vi "Day07-03_디지털 신호 제어.vi"() -> ()   [LabVIEW 2021]
uses:
  <vilib>/DAQmx/create/channels.llb/DAQmx Create Channel (DI-Digital Input).vi
  <vilib>/DAQmx/create/channels.llb/DAQmx Create Channel (DO-Digital Output).vi
  <vilib>/DAQmx/write.llb/DAQmx Write (Digital U8 1Chan 1Samp).vi
  <vilib>/DAQmx/read.llb/DAQmx Read (Digital 1D Bool 1Chan 1Samp).vi
  <vilib>/DAQmx/read.llb/DAQmx Read (Digital U8 1Chan 1Samp).vi
  <vilib>/DAQmx/read.llb/DAQmx Read (Analog 1D Wfm NChan NSamp).vi
  <vilib>/DAQmx/write.llb/DAQmx Write (Digital 1D Bool 1Chan 1Samp).vi
panel:
  in  "정지 3":bool
  in  "data 3":bool[](array[boolean]) caption="데이터"
  in  "정지 2":bool
  out "data 2":bool[](array[boolean]) caption="데이터"
  in  "정지":bool
  out "data":waveform(dbl)[](graph) caption="데이터"
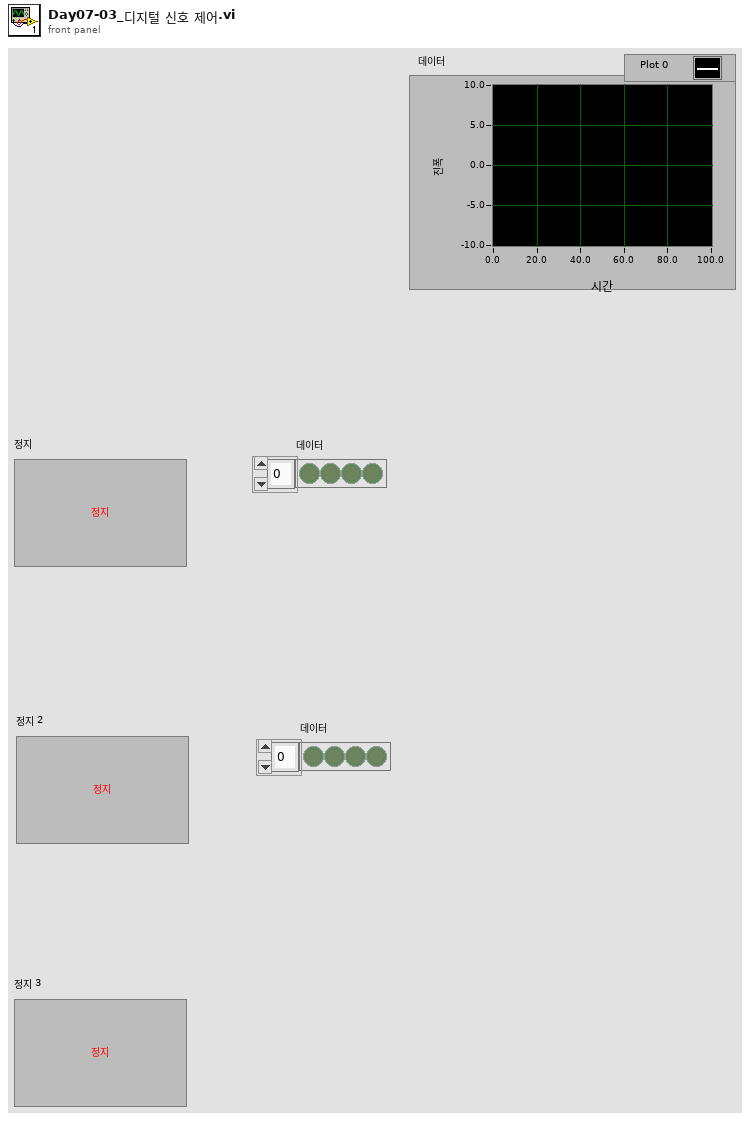
[diagram p1: front panel]
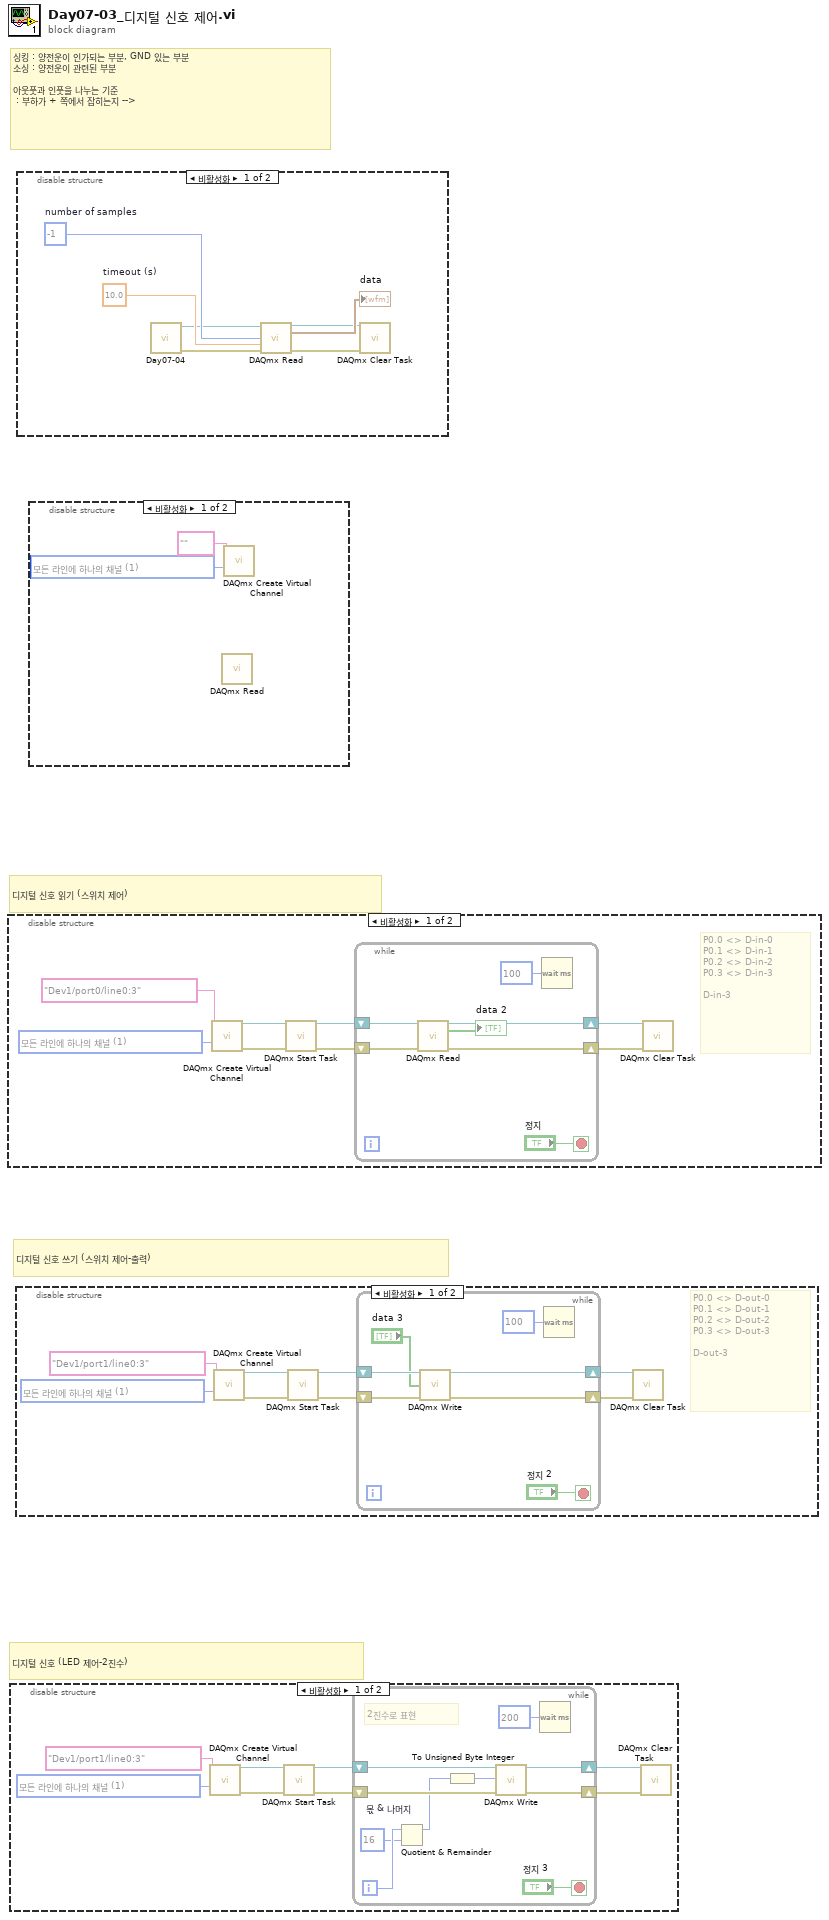
[diagram p0: block diagram]
diagram:
  # "디지털 신호 (LED 제어-2진수)"
  # "디지털 신호 쓰기 (스위치 제어-출력)"
  # "디지털 신호 읽기 (스위치 제어)"
  # "싱킹 : 양전운이 인가되는 부분, GND 있는 부분\n소싱 : 양전운이 관련된 부분\n\n아웃풋과 인풋을 나누는 기준\n : 부하가 + 쪽에서 잡히는지 -->"
  n1 = disable-structure shown="비활성화" {
    frame Disabled {
      w2 = 1 items=["각 라인에 하나의 채널", "모든 라인에 하나의 채널"] ("line grouping")
      # "P0.0 <> D-in-0\nP0.1 <> D-in-1\nP0.2 <> D-in-2\nP0.3 <> D-in-3\n\nD-in-3"
      n2 = call-poly <vilib>:"DAQmx Create Virtual Channel.vi"("lines"=tag "Dev1/port0/line0:3", "line grouping"=w2) -> ("task out"=w8:refnum<k21>, "error out"=w7:errorcluster)  [unwired: 12 in]
      n3 = call <vilib>:"DAQmx Start Task.vi"("task/channels in"=w8, "error in"=w7) -> ("task out"=w6:refnum<k21>, "error out"=w5:errorcluster)  [unwired: 12 in]
      n4 = while {
        shift-right: [w13] -> w4
        shift-left: w6 -> [w15]
        shift-right: [w12] -> w3
        shift-left: w5 -> [w14]
        stop <- "정지" stop-if-true
        n5 = call-poly <vilib>:"DAQmx Read.vi"("task/channels in"=w15, "error in"=w14) -> ("task out"=w13:refnum<k21>, "data"=→"data 2":bool[], "error out"=w12:errorcluster)  [unwired: 11 in]
        n6 = Wait (ms)(milliseconds to wait=u32 100 ("대기 시간 (ms)")) -> ()  [unwired: 1 out]
      }
      n7 = call <vilib>:"DAQmx Clear Task.vi"("task in"=w4, "error in"=w3) -> ()  [unwired: 13 in, 1 out]
    }
    frame Enabled {
    }
  }
  n8 = disable-structure shown="비활성화" {
    frame Disabled {
      w16 = 1 items=["각 라인에 하나의 채널", "모든 라인에 하나의 채널"] ("line grouping")
      n9 = call-poly <vilib>:"DAQmx Create Virtual Channel.vi"("lines"=tag "Dev1/port1/line0:3", "line grouping"=w16) -> ("task out"=w22:refnum<k21>, "error out"=w21:errorcluster)  [unwired: 12 in]
      n10 = call <vilib>:"DAQmx Start Task.vi"("task/channels in"=w22, "error in"=w21) -> ("task out"=w20:refnum<k21>, "error out"=w19:errorcluster)  [unwired: 12 in]
      n11 = while {
        shift-right: [w31] -> w18
        shift-left: w20 -> [w33]
        shift-right: [w30] -> w17
        shift-left: w19 -> [w32]
        i -> [w27]
        stop <- "정지 3" stop-if-true
        # "2진수로 표현"
        n12 = Quotient & Remainder "몫 & 나머지"(x=w27, y=16) -> (x-y*floor(x/y)=w25:i32)  [unwired: 1 out]
        n13 = To Unsigned Byte Integer(number=w25) -> (unsigned 8bit integer=w24:u8)
        n14 = call-poly <vilib>:"DAQmx Write.vi"("task/channels in"=w33, "data"=w24, "error in"=w32) -> ("task out"=w31:refnum<k21>, "error out"=w30:errorcluster)  [unwired: 10 in, 1 out]
        n15 = Wait (ms)(milliseconds to wait=u32 200 ("대기 시간 (ms)")) -> ()  [unwired: 1 out]
      }
      n16 = call <vilib>:"DAQmx Clear Task.vi"("task in"=w18, "error in"=w17) -> ()  [unwired: 13 in, 1 out]
    }
    frame Enabled {
    }
  }
  n17 = disable-structure shown="비활성화" {
    frame Disabled {
      w41 = 1 items=["각 라인에 하나의 채널", "모든 라인에 하나의 채널"] ("line grouping")
      # "P0.0 <> D-out-0\nP0.1 <> D-out-1\nP0.2 <> D-out-2\nP0.3 <> D-out-3\n\nD-out-3"
      n18 = call-poly <vilib>:"DAQmx Create Virtual Channel.vi"("lines"=tag "Dev1/port1/line0:3", "line grouping"=w41) -> ("task out"=w35:refnum<k21>, "error out"=w36:errorcluster)  [unwired: 12 in]
      n19 = call <vilib>:"DAQmx Start Task.vi"("task/channels in"=w35, "error in"=w36) -> ("task out"=w37:refnum<k21>, "error out"=w38:errorcluster)  [unwired: 12 in]
      n20 = while {
        shift-right: [w46] -> w39
        shift-left: w37 -> [w48]
        shift-right: [w45] -> w40
        shift-left: w38 -> [w47]
        stop <- "정지 2" stop-if-true
        n21 = call-poly <vilib>:"DAQmx Write.vi"("task/channels in"=w48, "data"="data 3", "error in"=w47) -> ("task out"=w46:refnum<k21>, "error out"=w45:errorcluster)  [unwired: 10 in, 1 out]
        n22 = Wait (ms)(milliseconds to wait=u32 100 ("대기 시간 (ms)")) -> ()  [unwired: 1 out]
      }
      n23 = call <vilib>:"DAQmx Clear Task.vi"("task in"=w39, "error in"=w40) -> ()  [unwired: 13 in, 1 out]
    }
    frame Enabled {
    }
  }
  n24 = disable-structure shown="비활성화" {
    frame Disabled {
      w53 = 10.0  # timeout (s)
      w54 = -1  # number of samples
      n25 = call "Day07-04.vi"() -> ("error out"=w49:errorcluster, "task out"=w50:refnum<k21>)  [unwired: 10 in]
      n26 = call-poly <vilib>:"DAQmx Read.vi"("task/channels in"=w50, "number of samples per channel"=w54, "timeout"=w53, "error in"=w49) -> ("task out"=w51:refnum<k21>, "data"=→"data":waveform(dbl)[], "error out"=w52:errorcluster)  [unwired: 9 in]
      n27 = call <vilib>:"DAQmx Clear Task.vi"("task in"=w51, "error in"=w52) -> ()  [unwired: 13 in, 1 out]
    }
    frame Enabled {
    }
  }
  n28 = disable-structure shown="비활성화" {
    frame Disabled {
      w57 = 1 items=["각 라인에 하나의 채널", "모든 라인에 하나의 채널"] ("line grouping")
      n29 = call-poly <vilib>:"DAQmx Read.vi"() -> ()  [unwired: 13 in, 3 out]
      n30 = call-poly <vilib>:"DAQmx Create Virtual Channel.vi"("lines"=tag "", "line grouping"=w57) -> ()  [unwired: 12 in, 2 out]
    }
    frame Enabled {
    }
  }
